vi "Initialize.vi"(8 "error in":errorcluster) -> (0 "error out":errorcluster, 3 "Messaging Structures":T1)   [LabVIEW 2020, in "Support.lvlib"]
doc: "Initializes project (messaging structures, database connection, ...)"
uses:
  Support.lvlib
  Controls/Project Messaging Structures.ctl
  Controls/Project Event Msg.ctl
  Controls/Project Events.ctl
  Error Handler/Controls/Error QMsg.ctl
  Controls/Project Modules.ctl
  Controller/Controls/Controller QMsg.ctl
  Controller/Controller.lvlib
  Error Handler/ErrorHandler.lvlib
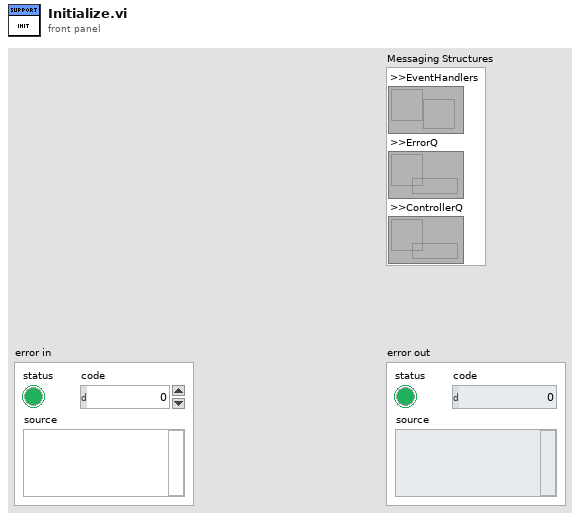
[diagram p1: front panel]
types:
  T1 = typedef "Support.lvlib/Project Messaging Structures.ctl" = cluster{">>EventHandlers":refnum<user-event>, ">>ErrorQ":refnum<queue>, ">>ControllerQ":refnum<queue>}
  T2 = typedef "ErrorHandler.lvlib/Error QMsg.ctl" = cluster{"Command":string, "Data":errorcluster, "Source Module":T3}
  T3 = typedef "Support.lvlib/Project Modules.ctl" = enum16{"Controller", "Error", "Configuration Database", "Sensor Interface", "User Console", "Display Console"}
  T4 = typedef "Controller.lvlib/Controller QMsg.ctl" = cluster{"Command":string, "Data":variant}
  T5 = typedef "Support.lvlib/Project Event Msg.ctl" = cluster{"Command":string, "Data":variant, "Events":T6}
  T6 = typedef "Support.lvlib/Project Events.ctl" = enum16{"Stop", "Initialize", "Elevator Call"}
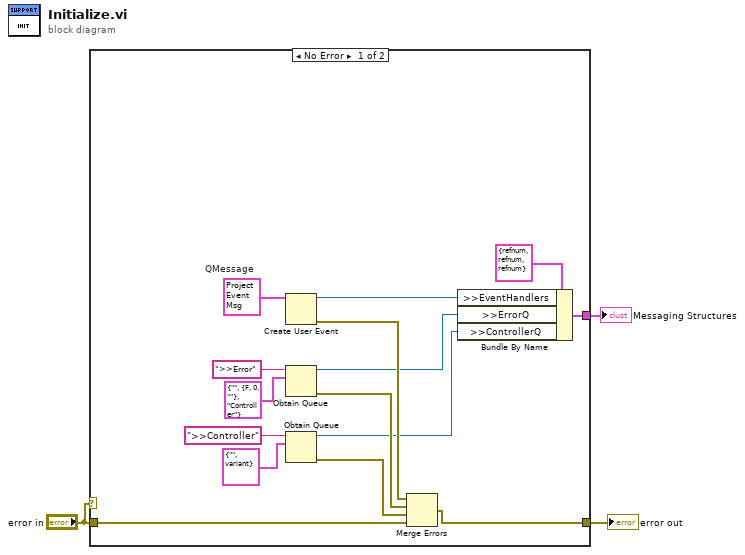
[diagram p0: block diagram]
diagram:
  n1 = case shown="No Error" "error in" {
    tunnel: "error in" -> [w10 w19]
    tunnel: [w9 w19] -> w2
    tunnel: [w7 _] -> w1
    frame No Error {
      w14 = T5 {"Command"="", "Data"=variant, "Events"=enum."Stop"}  # QMessage
      n2 = Create User Event(user event datatype=w14) -> (user event=w4:refnum<user-event>, error out=w13:errorcluster)  [unwired: 1 in]
      n3 = Obtain Queue(name (unnamed)=">>Error", element data type=T2 {"Command"="", "Data"={"status"=FALSE, "code"=0, "source"=""}, "Source Module"=enum."Controller"} ("QMessage")) -> (queue out=w5:refnum<queue>, error out=w12:errorcluster)  [unwired: 3 in, 1 out]
      n4 = Obtain Queue(name (unnamed)=">>Controller", element data type=T4 {"Command"="", "Data"=variant} ("QMessage")) -> (queue out=w6:refnum<queue>, error out=w11:errorcluster)  [unwired: 3 in, 1 out]
      n5 = Merge Errors(w13, w12, w11, w10) -> (w9:errorcluster)
      n6 = Bundle By Name(cluster=T1 {">>EventHandlers"=refnum, ">>ErrorQ"=refnum, ">>ControllerQ"=refnum} ("Messaging Structures"), ">>EventHandlers"=w4, ">>ErrorQ"=w5, ">>ControllerQ"=w6) -> (w7:T1)
    }
    frame Error {
    }
  }
  "error out" <- w2
  "Messaging Structures" <- w1
